vi "Single Channel Fetch Duty Cycle.vi"(8 "error in (no error)":errorcluster {"code" format="%.0x"}, 9 "LastPoint":i32 format="%.0g", 10 "FirstPoint":i32 format="%.0g", 11 "instrument handle":refnum<k15>) -> (0 "error out":errorcluster {"code" format="%.0x"}, 2 "Val":dbl, 3 "instrument handle out":refnum<k15>)   [LabVIEW 2020, in "Keysight DAQ970.lvlib"]
doc: "Performs post-processing calculation on the specified range of readings and returns duty cycle for single channel DMM digitizing."
uses:
  Keysight DAQ970.lvlib
  KtDAQ970.dll
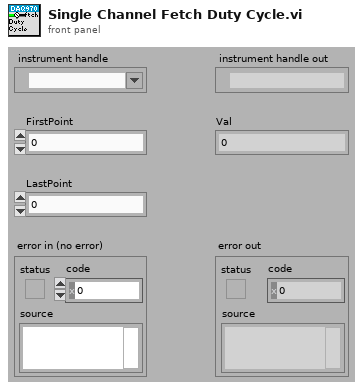
[diagram p1: front panel]
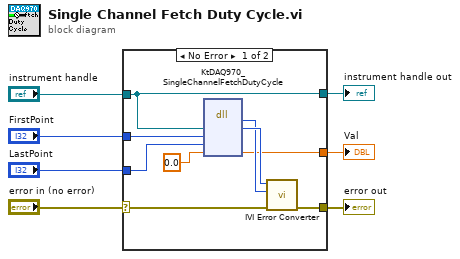
[diagram p0: block diagram]
diagram:
  n1 = case shown="No Error" "error in (no error)" {
    selector: "error in (no error)" -> [w14 w18]
    tunnel: [w13 w18] -> w7
    tunnel: "instrument handle" -> [w8 w17]
    tunnel: "FirstPoint" -> [w12 _]
    tunnel: "LastPoint" -> [w11 _]
    tunnel: [w9 _] -> w2
    tunnel: [w8 w17] -> w1
    frame No Error {
      n2 = dll-call lib="KtDAQ970**.dll" fn="KtDAQ970_SingleChannelFetchDutyCycle"("Vi"=w8, "FirstPoint"=w12, "LastPoint"=w11, "Val"=0.0) -> (w15:i32, "Vi"=w16:u32, "Val"=w9:dbl)  [unwired: 5 in, 2 out]
      n3 = call "IVI Error Converter.vi"("error in (no error)"=w14, "IVI error code (0)"=w15, "instrument handle"=w16) -> ("error out"=w13:errorcluster)  [unwired: 7 in, 1 out]
    }
    frame Error {
    }
  }
  "error out" <- w7
  "instrument handle out" <- w1
  "Val" <- w2
